vi "LH6ResponseACK_inycom.vi"(8 "error in":errorcluster, 11 "Response in":string[](array[string])) -> (0 "error out":errorcluster, 3 "Response  out":string[](array[string]))   [LabVIEW 2015]
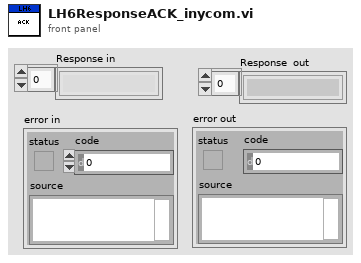
[diagram p1: front panel]
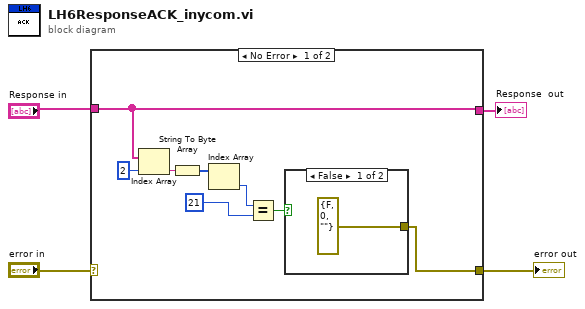
[diagram p0: block diagram]
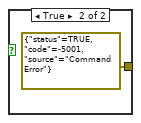
[diagram p2: hidden frame]
diagram:
  n1 = case shown="No Error" "error in" {
    selector: "error in" -> [_ w16]
    tunnel: "Response in" -> [w5 w15]
    tunnel: [w6 w16] -> w2
    tunnel: [w5 w15] -> w1
    frame No Error {
      n2 = Index Array(array=w5, index=2) -> (element=w11:string)
      n3 = String To Byte Array(string=w11) -> (unsigned byte array=w9:u8[])
      n4 = Index Array(array=w9) -> (element=w8:u8)  [unwired: 1 in]
      n5 = Equal?(x=w8, y=u8 21) -> (x = y?=w12:bool)
      n6 = case shown="False" w12 {
        tunnel: [errorcluster {"status"=FALSE, "code"=0, "source"=""} ("error IO") errorcluster {"status"=TRUE, "code"=-5001, "source"="Command Error"} ("error IO")] -> w6
        frame False {
        }
        frame True {
        }
      }
    }
    frame Error {
    }
  }
  "error out" <- w2
  "Response  out" <- w1
